vi "Change Format String.vi"(8 "error in (no error)":errorcluster, 10 "Format String":string caption="Time Type", 11 "Numeric Data Type in":refnum<class "Numeric Data Type.lvclass">) -> (0 "error out":errorcluster, 3 "Numeric Data Type out":refnum<class "Numeric Data Type.lvclass">)   [LabVIEW 2018, in "Numeric Data Type.lvclass"]
uses:
  Numeric Data Type.lvclass
  Numeric Data Type.lvclass/Numeric Data Type.ctl
  Reference Valid.vi
  Reference Revert.vi
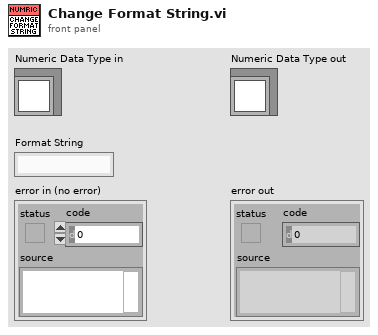
[diagram p1: front panel]
types:
  T1 = enum8{"Enabled", "Disabled", "Disabled and Grayed Out"}
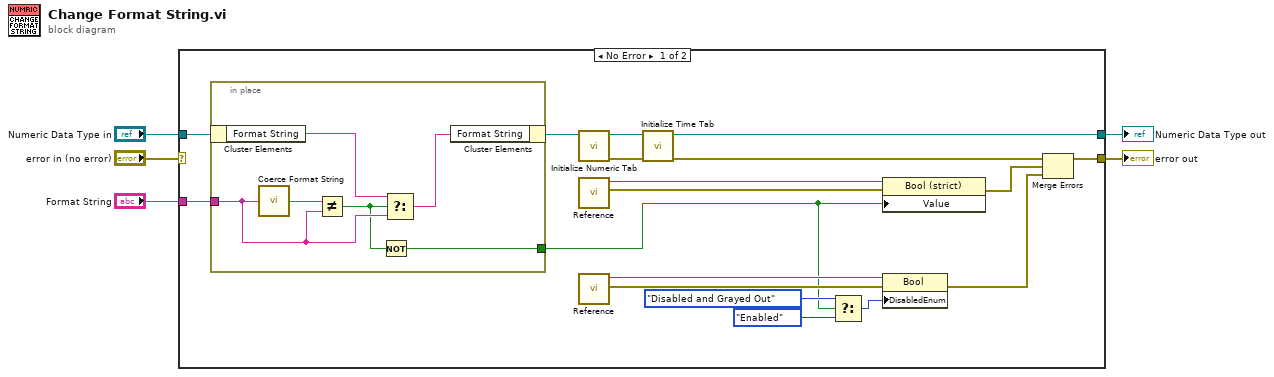
[diagram p0: block diagram]
diagram:
  n1 = case shown="No Error" "error in (no error)" {
    selector: "error in (no error)" -> [_ w31]
    tunnel: [w11 w31] -> w4
    tunnel: [w22 w30] -> w2
    tunnel: "Numeric Data Type in" -> [w23 w30]
    tunnel: "Format String" -> [w20 _]
    frame No Error {
      n2 = in-place {
        in-place-border: w20 -> [w28]
        in-place-border: [w24] -> w14
        n3 = in-place-cluster #1(w23) -> ("Format String"=w27:string)
        n4 = call "Coerce Format String.vi"("Format String"=w28) -> ("Coerced String"=w29:string)
        n5 = Not Equal?(x=w29, y=w28) -> (x != y?=w25:bool)
        n6 = Not(x=w25) -> (.not. x?=w24:bool)
        n7 = Select(t=w27, s=w25, f=w28) -> (s? t:f=w26:string)
        n8 = in-place-cluster #1("Format String"=w26) -> (w8:refnum<class "Numeric Data Type.lvclass">)
      }
      n9 = call "Initialize Numeric Tab.vi"("Numeric Data Type in"=w8) -> ("error out"=w6:errorcluster, "Numeric Data Type (dub)"=w7:refnum<class "Numeric Data Type.lvclass">)  [unwired: 9 in]
      n10 = call-poly "Reference.vi"() -> ("error out"=w18:errorcluster, "Valid"=w19:refnum<vi>)  [unwired: 10 in]
      n11 = call-poly "Reference.vi"() -> ("error out"=w16:errorcluster, "Revert"=w17:refnum<vi>)  [unwired: 10 in]
      n12 = call "Initialize Time Tab.vi"("error in (no error)"=w6, "Numeric Data Type in"=w7) -> ("error out"=w21:errorcluster, "Numeric Data Type (dub)"=w22:refnum<class "Numeric Data Type.lvclass">)  [unwired: 8 in]
      n13 = Select(t=T1."Disabled and Grayed Out" ("Disabled"), s=w14, f=T1."Enabled" ("Disabled")) -> (s? t:f=w12:T1)
      n14 = property class="Bool (strict)"(reference=w19, error in=w18, "Value"=w14) -> (error out=w10:errorcluster)  [unwired: 1 out]
      n15 = property class="Bool"(reference=w17, error in=w16, "DisabledEnum"=w12) -> (error out=w9:errorcluster)  [unwired: 1 out]
      n16 = Merge Errors(w21, w10, w9) -> (w11:errorcluster)
    }
    frame Error {
    }
  }
  "error out" <- w4
  "Numeric Data Type out" <- w2
